vi "Send Select Display Mode.vi"(7 "Message Priority (Normal)":T2=enum."Normal", 8 "error in (no error)":errorcluster, 10 "DisplayMode":T1, 11 "Message Enqueuer":refnum<class "Message Enqueuer.lvclass">) -> (0 "error out":errorcluster, 3 "Message Enqueuer out":refnum<class "Message Enqueuer.lvclass">)   [LabVIEW 2023, in "Instruments.lvlib" / "Select Display Mode Msg.lvclass"]
doc: "This VI sends the message to an actor."
uses:
  Select Display Mode Msg.lvclass
  builds/Framework/Actor Framework.lvlibp/1abvi3w/vi.lib/ActorFramework/Message Enqueuer/Message Enqueuer.lvclass
  builds/Framework/Actor Framework.lvlibp/1abvi3w/vi.lib/ActorFramework/Message Enqueuer/Message Priority.ctl
  Custom Controls/Display Mode.ctl
  Select Display Mode Msg.lvclass/Select Display Mode Msg.ctl
  C:/Users/Public/Documents/Development/builds/Framework/Actor Framework.lvlibp/1abvi3w/vi.lib/ActorFramework/Message/Message.lvclass
  Library/Instruments.lvclass
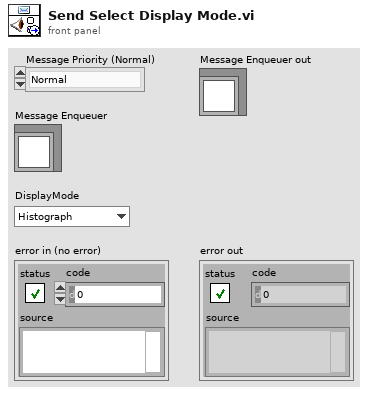
[diagram p1: front panel]
types:
  T1 = typedef "Instruments.lvlib/Instruments.lvclass/Display Mode.ctl" = enum16{"Histograph", "Table", "Snapshot"}
  T2 = typedef "Actor Framework.lvlibp/Message Enqueuer.lvclass/Message Priority.ctl" = enum16{"Low", "Normal", "High"}
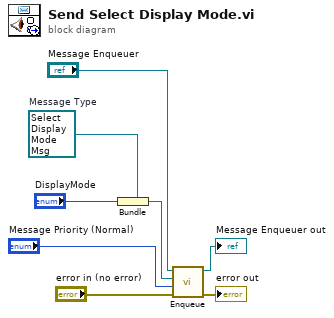
[diagram p0: block diagram]
diagram:
  w5 = refnum<class "Select Display Mode Msg.lvclass"> refnum  # Message Type
  n1 = Bundle(cluster=w5, "DisplayMode") -> (w4:refnum<class "Select Display Mode Msg.lvclass">)
  n2 = call "Enqueue.vi"("error in (no error)"="error in (no error)", "Message Priority (Normal)"="Message Priority (Normal)", "Message"=w4, "Message Enqueuer in"="Message Enqueuer") -> ("error out"=→"error out":errorcluster, "Message Enqueuer out"=→"Message Enqueuer out":refnum<class "Message Enqueuer.lvclass">)  [unwired: 6 in]
